vi "PH_Beamline.color Booster BL.vi"(0 "i ref in":refnum<vi>, 2 "Color State Booster Input":i32, 5 "error in (no error)":errorcluster) -> (14 "i ref out":refnum<vi>, 16 "Color State Booster Exit to MT":i32, 17 "Color State Booster Exit to Compressor":i32, 19 "error out":errorcluster)   [LabVIEW 2014, in "PH_Beamline.lvlib"]
doc: "This Vi colors the Booster beamline elements."
uses:
  PH_Beamline.lvlib
  PH_Basics/PH_StatusHandler/PH_StatusHandler.Status.ctl
  PH_Basics/PH_Common/PH_Common.lvlib
  PH_BL-Master/PH_BL-Master.lvlib
  PH_Basics/PH_StatusHandler/PH_StatusHandler.lvlib
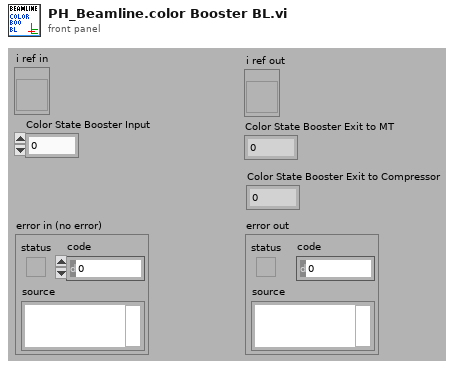
[diagram p1: front panel]
types:
  T1 = typedef "PH_StatusHandler.lvlib/PH_StatusHandler.Status.ctl" = i16
  T2 = typedef "PH_Beamline.lvlib/PH_Beamline.i attribute.ctl" = cluster{"GUI Refs":cluster{"PA ok":refnum<vi>, "MA ok":refnum<vi>, "fs FE ok":refnum<vi>, "ns FE ok":refnum<vi>, "PA ED ok":refnum<vi>, "MAS ok":refnum<vi>, "Booster ok":refnum<vi>, "Mirrortower ok":refnum<vi>, "In.-Box ok":refnum<vi>, "Compressor ok":refnum<vi>, "Experiment LB ok":refnum<vi>, "Experiment LL ok":refnum<vi>, "PHELIX_Beckhoff_Watchdog":refnum<vi>, "Shutters closed":refnum<vi>, "uOPA ok":refnum<vi>, "Vacuum no shotcond Comp LB":refnum<vi>}, "Refs BL MA":refnum<vi>[], "Refs BL MA-IB":refnum<vi>[], "Refs BL fs":refnum<vi>[], "Refs BL PA ED":refnum<vi>[], "Refs BL MAS":refnum<vi>[], "Refs BL Boo":refnum<vi>[], "Refs BL ns":refnum<vi>[], "Refs BL Mirrortower":refnum<vi>[], "Refs BL Compressor":refnum<vi>[], "Refs BL Exp LB":refnum<vi>[], "Radiation Safety":cluster{"Exp Laserbay":cluster{"Ref Op Mode":refnum<vi>, "Ref Laserbay evacuated":refnum<vi>, "Tagname LB evacuated":string, "Shot Mode":T3, "Laserbay evacuated?":i32, "Tagname HV room locked":string, "HV room locked?":i32, "Ref HV room locked":refnum<vi>, "Tagname bridged?":string, "Ref Bridge":refnum<vi>, "I<1E18W/cm²":bool}, "Exp Laserlab":cluster{"Ref Op Mode":refnum<vi>, "Ref Laserlab evacuated":refnum<vi>, "Tagname LL evacuated":string, "Shot Mode":T3, "Laserlab evacuated?":i32, "Tagname bridged?":string, "Ref Bridge":refnum<vi>, "I<1E18W/cm²":bool}}, "Refs BL LL":refnum<vi>[], "PP Igni Heating GUI Refs":refnum<vi>[], "PP Igni Heating Tagnames ":string[], "Refs BL PA":cluster{"undelayed Line before Shutter":refnum<vi>[], "undelayed Line after Shutter":refnum<vi>[], "before Bypass":refnum<vi>[], "delayed Line before Shutter":refnum<vi>[], "delayed Line after Shutter":refnum<vi>[], "before Shutter Input":refnum<vi>[], "after Shutter Input":refnum<vi>[], "Bypass":refnum<vi>[], "before Shutter Exit":refnum<vi>[], "after Shutter Exit":refnum<vi>[], "to MA":refnum<vi>[], "to Lab":refnum<vi>[]}, "BL":cluster{"YLF_BL_Status":i32, "fs_BL_Status":i32, "fs_YLF_BL_Status":i32, "ns_BL_Status":i32, "PA_Input_BL_Status":i32, "PA_UnDelay_BL_Status":i32, "PA_Delay_BL_Status":i32, "PA_BL_Status":i32, "PA_Bypass_BL_Status":i32, "PA_Exit_BL_Status":i32, "PA_LL_BL_Status":i32, "LL_BL_Status":i32, "PA_MA_BL_Status":i32, "MA_Exit_BL_Status":i32, "MA_Z6_BL_Status":i32, "Z6_BL_Status":i32, "MA_LB_BL_Status":i32, "LB_TB2_BL_Status":i32, "PA_before_Bypass_BL_Status":i32, "LB_TB3_BL_Status":i32}, "State Subsystems":cluster{"PA":bool, "MA":bool, "ns FE":bool, "fs FE":bool, "PA ED":bool, "In.-Box":bool, "MAS":bool, "Booster":bool, "Mirrortower":bool, "Compressor":bool, "Experiment LB":bool, "Experiment LL":bool, "uOPA":bool}, "Status Subscriber Information":T4, "Refs BL uOPA":refnum<vi>[], "PA_Input_2_Beam_6PWpGUI not linked?":bool, "PA_Input_Delay_6PGUI not linked?":bool, "Settings":T7}
  T3 = typedef "PH_Beamline.lvlib/PH_Beamline.Operation Mode.ctl" = i32
  T4 = typedef "PH_Beamline.lvlib/PH_Beamline.Status Subscriber Information.ctl" = cluster{"fs Swich YLF":T5, "fs Exit Shutter":T5, "ns Exit Shutter":T5, "PA Input Shutter":T5, "PA PC WP":T5, "PA PC WP 2":T5, "PA Bypass In":T5, "PA Bypass Out":T5, "PA CH 1":T5, "PA delayed":T5, "PA non delayed":T5, "PA Exit Shutter":T5, "PA Switch Lab":T5, "PA Bridge CH Input MA":T5, "MA Diffusor IB":T5, "MA IB Ready":T5, "MA CH 1":T5, "MA CH 2":T5, "MA CH 3":T5, "MA CH 4":T5, "MA Shutter Align Cam":T5, "MA Position MM5":T5, "Calorimeter Switch":T5, "BL Z6 CH 9":T5, "BL Z6 Beamdump":T5, "BL Z6 Shutter":T5, "COS Sensitivity Switch":T5, "Exp LB Shutter":T5, "Exp LB TB 2":T5, "Exp LB TB 3":T5, "PA LL Input CH":T5, "PA LL Output CH":T5, "LL Comp Input Shutter":T5, "LL Comp Output Shutter":T5, "LL Comp FF Shutter":T5, "Exp LL Shutter":T5, "MA IM In IB":T5, "MA IM Out IB":T5, "MA DB In IB":T5, "MA DB Out IB":T5, "Exp LB Shutter Interlock":T5, "Exp LL Shutter Interlock":T5, "MM1 Force Sensor":T5}
  T5 = typedef "PH_BL-Master.lvlib/PH_BL-Master.Status Subscriber Information.ctl" = cluster{"Index of element":i32, "Attributeset":T6}
  T6 = typedef "PH_BL-Master.lvlib/PH_BL-Master.Attribute Set.ctl" = enum16{"Boolean Status Service Subscriber", "Picture Status Service Subscriber"}
  T7 = typedef "PH_Beamline_Chief.lvlib/PH_Beamline_Chief.Settings.ctl" = cluster{"PA Doublepass Mode":bool, "Compressor Vaccuum LB not relevant":bool, "Windowshutter TB2 not relevant":bool, "Windowshutter TB3 not relevant":bool}
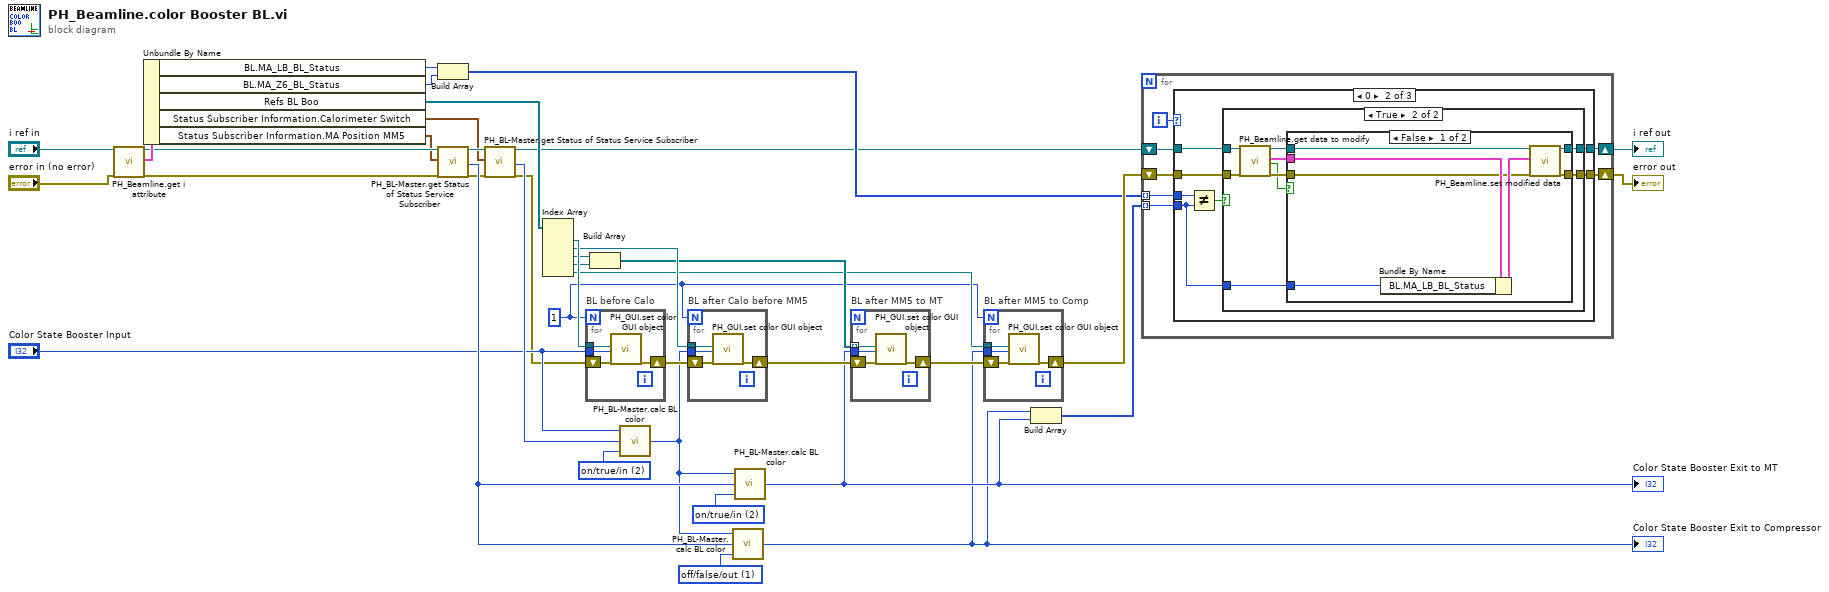
[diagram p0: block diagram]
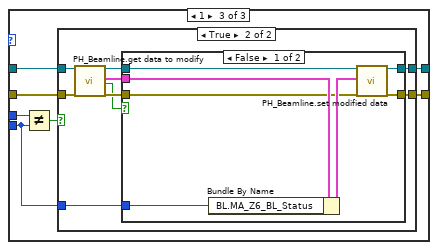
[diagram p5: hidden frame]
diagram:
  w13 = T1 2 items=["no info", "off/false/out", "on/true/in", "Failure", "Alarm", "Status 1", "Status 2", "Status 3"] ("State for \"2\" (on) of ABLE (off/false/out)")
  w14 = T1 2 items=["no info", "off/false/out", "on/true/in", "Failure", "Alarm", "Status 1", "Status 2", "Status 3"] ("State for \"2\" (on) of ABLE (off/false/out)")
  w15 = T1 1 items=["no info", "off/false/out", "on/true/in", "Failure", "Alarm", "Status 1", "Status 2", "Status 3"] ("State for \"2\" (on) of ABLE (off/false/out)")
  w9 = 1
  n1 = call "PH_Beamline.get i attribute.vi"("i ref in"="i ref in", "error in (no error)"="error in (no error)") -> ("i ref out"=w5:refnum<vi>, "i attribute"=w38:T2, "error out"=w6:errorcluster)  [unwired: 15 in]
  n2 = Unbundle By Name(w38) -> ("BL.MA_LB_BL_Status"=w17:i32, "BL.MA_Z6_BL_Status"=w18:i32, "Refs BL Boo"=w37:refnum<vi>[], "Status Subscriber Information.Calorimeter Switch"=w2:T5, "Status Subscriber Information.MA Position MM5"=w1:T5)
  n3 = Build Array(w17, w18) -> (w16:i32[])
  n4 = call "PH_BL-Master.get Status of Status Service Subscriber.vi"("i ref in"=w5, "Wanted Status Subscriber Information"=w1, "error in (no error)"=w6) -> ("i ref out"=w12:refnum<vi>, "Status"=w28:T1, "error out"=w11:errorcluster)  [unwired: 11 in, 3 out]
  n5 = call "PH_BL-Master.get Status of Status Service Subscriber.vi"("i ref in"=w12, "Wanted Status Subscriber Information"=w2, "error in (no error)"=w11) -> ("i ref out"=w3:refnum<vi>, "Status"=w29:T1, "error out"=w4:errorcluster)  [unwired: 11 in, 3 out]
  n6 = Index Array(array=w37) -> (element #1=w36:refnum<vi>, element #2=w35:refnum<vi>, element #3=w34:refnum<vi>, element #4=w33:refnum<vi>, element #5=w30:refnum<vi>)  [unwired: 5 in]
  n7 = for "BL before Calo" {
    N: w9 -> [_]
    tunnel: w36 -> [w42]
    shift-right: [w40] -> w27
    shift-left: w4 -> [w41]
    tunnel: "Color State Booster Input" -> [w39]
    n8 = call "PH_GUI.set color GUI object.vi"("GUI object Ref"=w42, "State"=w39, "error in (no error)"=w41) -> ("error out"=w40:errorcluster)  [unwired: 16 in]
  }
  n9 = Build Array(w34, w33) -> (w32:refnum<vi>[])
  n10 = call "PH_BL-Master.calc BL color.vi"("State for \"2\" (on) of ABLE (off/false/out)"=w14, "State ABLE"=w29, "State before ABLE"="Color State Booster Input") -> ("State after ABLE"=w25:i32)
  n11 = for "BL after Calo before MM5" {
    N: w9 -> [_]
    tunnel: w35 -> [w46]
    shift-right: [w44] -> w26
    shift-left: w27 -> [w45]
    tunnel: w25 -> [w43]
    n12 = call "PH_GUI.set color GUI object.vi"("GUI object Ref"=w46, "State"=w43, "error in (no error)"=w45) -> ("error out"=w44:errorcluster)  [unwired: 16 in]
  }
  n13 = call "PH_BL-Master.calc BL color.vi"("State for \"2\" (on) of ABLE (off/false/out)"=w15, "State ABLE"=w28, "State before ABLE"=w25) -> ("State after ABLE"=w20:i32)
  "Color State Booster Exit to Compressor" <- w20
  n14 = call "PH_BL-Master.calc BL color.vi"("State for \"2\" (on) of ABLE (off/false/out)"=w13, "State ABLE"=w28, "State before ABLE"=w25) -> ("State after ABLE"=w21:i32)
  "Color State Booster Exit to MT" <- w21
  n15 = for "BL after MM5 to MT" {
    tunnel: w32 -> [w50] mode=indexing
    shift-right: [w48] -> w31
    shift-left: w26 -> [w49]
    tunnel: w21 -> [w47]
    n16 = call "PH_GUI.set color GUI object.vi"("GUI object Ref"=w50, "State"=w47, "error in (no error)"=w49) -> ("error out"=w48:errorcluster)  [unwired: 16 in]
  }
  n17 = for "BL after MM5 to Comp" {
    N: w9 -> [_]
    tunnel: w30 -> [w54]
    shift-right: [w52] -> w23
    shift-left: w31 -> [w53]
    tunnel: w20 -> [w51]
    n18 = call "PH_GUI.set color GUI object.vi"("GUI object Ref"=w54, "State"=w51, "error in (no error)"=w53) -> ("error out"=w52:errorcluster)  [unwired: 16 in]
  }
  n19 = Build Array(w20, w21) -> (w19:i32[])
  n20 = for {
    shift-right: [w60] -> w22
    shift-left: w23 -> [w61]
    tunnel: w19 -> [w56] mode=indexing
    tunnel: w16 -> [w57] mode=indexing
    shift-right: [w58] -> w10
    shift-left: w3 -> [w59]
    i -> [w55]
    n21 = case shown="0" w55 {
      tunnel: [w62 w69 w96] -> w60
      tunnel: w61 -> [w62 w68 w95]
      tunnel: [w63 w67 w94] -> w58
      tunnel: w59 -> [w63 w66 w93]
      tunnel: w56 -> [_ w65 w92]
      tunnel: w57 -> [_ w64 w91]
      frame Default {
      }
      frame 0 {
        n22 = Not Equal?(x=w64, y=w65) -> (x != y?=w70:bool)
        n23 = case shown="True" w70 {
          tunnel: w66 -> [w72 w77]
          tunnel: [w72 w76] -> w67
          tunnel: w68 -> [w71 w75]
          tunnel: [w71 w74] -> w69
          tunnel: w65 -> [_ w73]
          frame False {
          }
          frame True {
            n24 = call "PH_Beamline.get data to modify.vi"("i ref in"=w77, "error in (no error)"=w75) -> ("i ref out"=w80:refnum<vi>, "i attribute"=w78:T2, "timed out"=w79:bool, "error out"=w81:errorcluster)  [unwired: 14 in]
            n25 = case shown="False" w79 {
              tunnel: w81 -> [w82 w89]
              tunnel: w80 -> [w88 w90]
              tunnel: [w87 w89] -> w74
              tunnel: [w86 w90] -> w76
              tunnel: w78 -> [w83 _]
              tunnel: w73 -> [w84 _]
              frame False {
                n26 = Bundle By Name(cluster=w83, "BL.MA_LB_BL_Status"=w84) -> (w85:T2)
                n27 = call "PH_Beamline.set modified data.vi"("i ref in"=w88, "i attribute"=w85, "error in (no error)"=w82) -> ("i ref out"=w86:refnum<vi>, "error out"=w87:errorcluster)  [unwired: 15 in]
              }
              frame True {
              }
            }
          }
        }
      }
      frame 1 {
        n28 = Not Equal?(x=w91, y=w92) -> (x != y?=w97:bool)
        n29 = case shown="True" w97 {
          tunnel: w93 -> [w99 w104]
          tunnel: [w99 w103] -> w94
          tunnel: w95 -> [w98 w102]
          tunnel: [w98 w101] -> w96
          tunnel: w92 -> [_ w100]
          frame False {
          }
          frame True {
            n30 = call "PH_Beamline.get data to modify.vi"("i ref in"=w104, "error in (no error)"=w102) -> ("i ref out"=w107:refnum<vi>, "i attribute"=w105:T2, "timed out"=w106:bool, "error out"=w108:errorcluster)  [unwired: 14 in]
            n31 = case shown="False" w106 {
              tunnel: w108 -> [w109 w116]
              tunnel: w107 -> [w115 w117]
              tunnel: [w114 w116] -> w101
              tunnel: [w113 w117] -> w103
              tunnel: w105 -> [w110 _]
              tunnel: w100 -> [w111 _]
              frame False {
                n32 = Bundle By Name(cluster=w110, "BL.MA_Z6_BL_Status"=w111) -> (w112:T2)
                n33 = call "PH_Beamline.set modified data.vi"("i ref in"=w115, "i attribute"=w112, "error in (no error)"=w109) -> ("i ref out"=w113:refnum<vi>, "error out"=w114:errorcluster)  [unwired: 15 in]
              }
              frame True {
              }
            }
          }
        }
      }
    }
  }
  "error out" <- w22
  "i ref out" <- w10
